vi "Read right terminal.vi"(9 "FlatSequenceInnerTunnel in":refnum<class "FlatSequenceInnerTunnel.lvclass">) -> (3 "FlatSequenceInnerTunnel out":refnum<class "FlatSequenceInnerTunnel.lvclass">, 4 "right terminal":refnum<class "Terminal.lvclass">)   [LabVIEW 2014, in "Raspberry Pi Compatible Compiler for LabVIEW.lvlib" / "FlatSequenceInnerTunnel.lvclass"]
uses:
  FlatSequenceInnerTunnel.lvclass
  Terminal/Terminal.lvclass
  FlatSequenceInnerTunnel.lvclass/FlatSequenceInnerTunnel.ctl
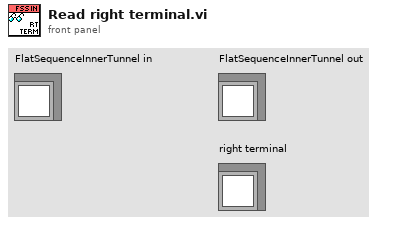
[diagram p1: front panel]
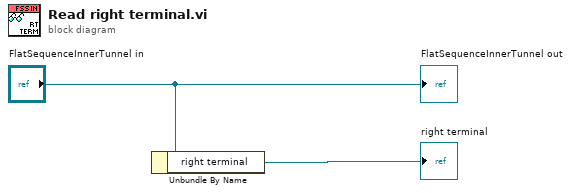
[diagram p0: block diagram]
diagram:
  n1 = Unbundle By Name("FlatSequenceInnerTunnel in") -> ("right terminal"=→"right terminal":refnum<class "Terminal.lvclass">)
  "FlatSequenceInnerTunnel out" <- "FlatSequenceInnerTunnel in"
